vi "WPI_DashboardNTL FF to New Position2.vi"(7 "Version":i32=2, 8 "VI Refnum":refnum<vi>, 10 "TimeOffset (s)":dbl, 11 "Byte Stream File in":refnum<file>) -> (0 "Strings":T1, 1 "Unchanged":bool, 2 "New time (s)":dbl, 3 "Byte Stream File out":refnum<file>)   [LabVIEW 2025]
uses:
  <vilib>/Rock Robotics/WPI/Dashboard/WPI_DashboardLoggingRecord.ctl
  <vilib>/Rock Robotics/WPI/Dashboard/WPI_DashboardLogging Global.vi
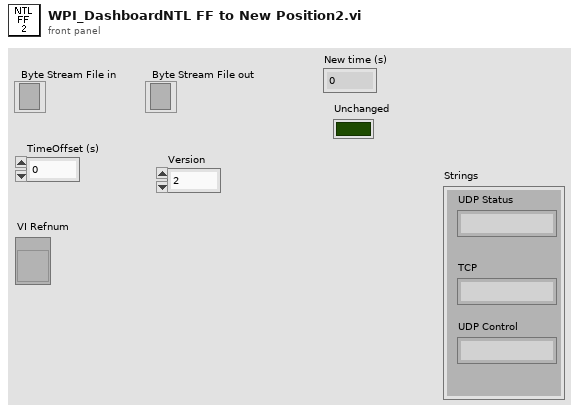
[diagram p1: front panel]
types:
  T1 = cluster{"UDP Status":string, "TCP":string, "UDP Control":string}
  T2 = typedef "WPI_DashboardLoggingRecord.ctl" = cluster{"time Ofst":i32, "video index":i32, "video index 2":i32, "video index 3":i32, "video index 4":i32, "UDP Status":string, "TCP":string, "UDP Control":string, "NT Updates":variant[]}
  T3 = cluster{"video index":i32, "video index 2":i32, "video index 3":i32, "video index 4":i32}
  T4 = cluster{"Video 1":i32, "Video 2":i32, "Video 3":i32, "Video 4":i32}
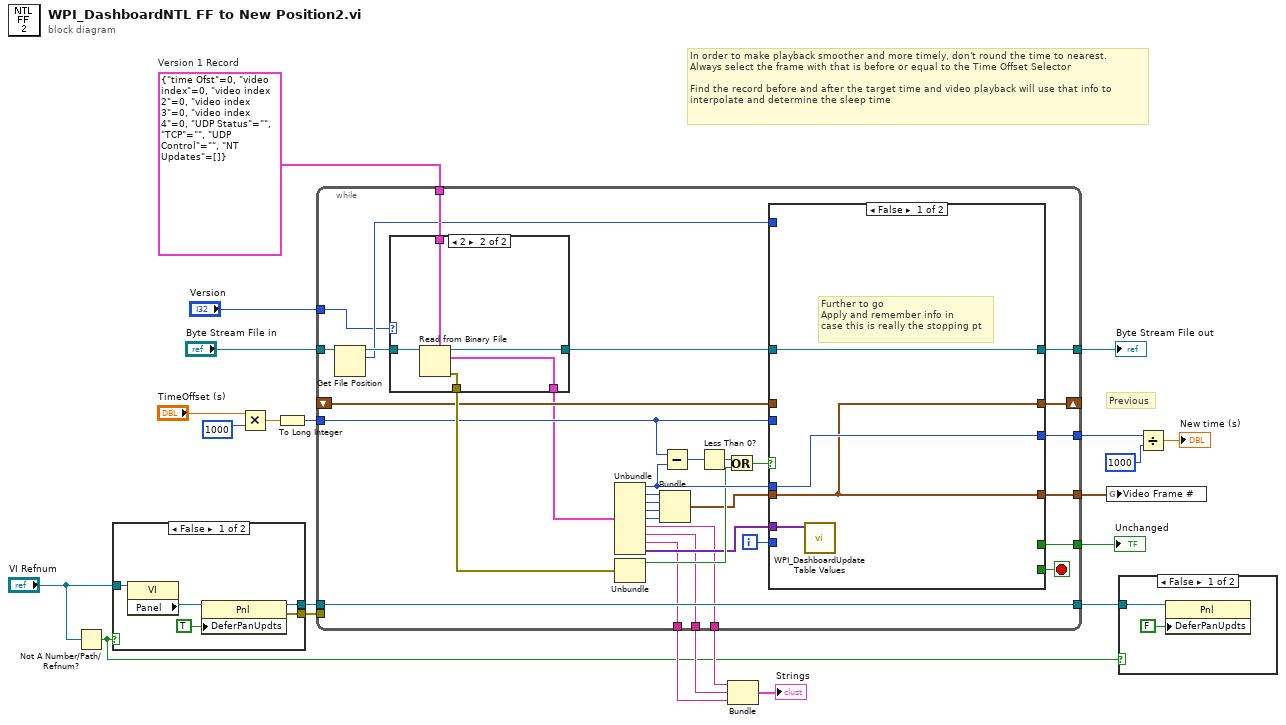
[diagram p0: block diagram]
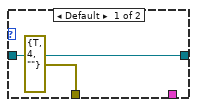
[diagram p4: hidden frame]
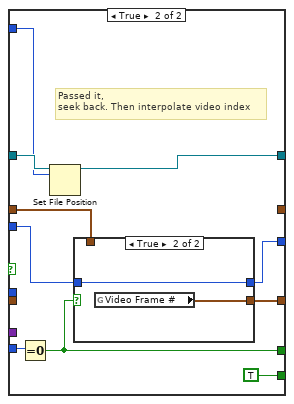
[diagram p5: hidden frame]
diagram:
  w4 = T2 {"time Ofst"=0, "video index"=0, "video index 2"=0, "video index 3"=0, "video index 4"=0, "UDP Status"="", "TCP"="", "UDP Control"="", "NT Updates"=[]}  # Version 1 Record
  # "Previous"
  # "In order to make playback smoother and more timely, don't round the time to nearest.\nAlways select the frame with that is before or equal to the Time Offset Selector\n\nFind the record before and after the target time and video playback will use that info to\ninterpolate and determine the sleep time"
  n1 = Not A Number/Path/Refnum?(number/path/refnum="VI Refnum") -> (NaN/Path/Refnum?=w1:bool)
  n2 = case shown="False" w1 {
    tunnel: [w25 _] -> w10
    tunnel: [w24 _] -> w9
    tunnel: "VI Refnum" -> [w23 _]
    frame False {
      n3 = property class="VI"(reference=w23) -> ("Panel"=w27:refnum<vi>)  [unwired: 1 in, 2 out]
      n4 = property class="Pnl"(reference=w27, "DeferPanUpdts"=TRUE ("Defer Panel Updates")) -> (reference out=w25:refnum<vi>, error out=w24:errorcluster)  [unwired: 1 in]
    }
    frame True {
    }
  }
  n5 = Multiply(x="TimeOffset (s)", y=1000) -> (x*y=w17:dbl)
  n6 = To Long Integer(number=w17) -> (32bit integer=w16:i32)
  n7 = while {
    tunnel: w4 -> [w59]
    tunnel: "Byte Stream File in" -> [w46]
    tunnel: [w56] -> w21
    tunnel: w16 -> [w52]
    shift-right: [w55] -> _
    shift-left: _ -> [w54]
    tunnel: [w50] -> w20
    tunnel: [w48] -> w13
    tunnel: [w47] -> w12
    tunnel: [w34] -> w8
    tunnel: [w36] -> w7
    tunnel: w10 -> [w38]
    tunnel: [w38] -> w11
    tunnel: w9 -> [_]
    tunnel: [w35] -> w6
    tunnel: "Version" -> [w28]
    i -> [w49]
    stop <- w39 stop-if-true
    n8 = Get File Position(7:w46) -> (2:w44:i64, 3:w45:refnum<file>)  [unwired: 1 in, 1 out]
    n9 = case shown="2" w28 {
      tunnel: w59 -> [_ w66]
      tunnel: [errorcluster {"status"=TRUE, "code"=4, "source"=""} ("error constant") w65] -> w58
      tunnel: [w60 w64] -> w57
      tunnel: [_ w63] -> w51
      tunnel: w45 -> [w60 w62]
      frame Default {
      }
      frame 2 {
        n10 = Read from Binary File(5:w66, 11:w62) -> (0:w65:errorcluster, 2:w63:T2, 3:w64:refnum<file>)  [unwired: 4 in, 1 out]
      }
    }
    n11 = Unbundle(w51) -> ("time Ofst"=w53:i32, "video index"=w33:i32, "video index 2"=w32:i32, "video index 3"=w31:i32, "video index 4"=w30:i32, "UDP Status"=w34:string, "TCP"=w35:string, "UDP Control"=w36:string, "NT Updates"=w37:variant[])
    n12 = Unbundle(w58) -> ("status"=w40:bool)  [unwired: 2 out]
    n13 = Bundle("video index"=w33, "video index 2"=w32, "video index 3"=w31, "video index 4"=w30) -> (w29:T3)  [unwired: 1 in]
    n14 = Subtract(x=w52, y=w53) -> (x-y=w41:i32)
    n15 = Less Than 0?(x=w41) -> (x < 0?=w43:bool)
    n16 = Or(x=w43, y=w40) -> (x .or. y?=w42:bool)
    n17 = case shown="False" w42 {
      tunnel: w57 -> [w69 w79]
      tunnel: [w69 w78] -> w56
      tunnel: [w67 _] -> w55
      tunnel: w54 -> [_ w71]
      tunnel: [_ TRUE] -> w39
      tunnel: w53 -> [w70 _]
      tunnel: w52 -> [_ w72]
      tunnel: w37 -> [w68 _]
      tunnel: [w70 w74] -> w50
      tunnel: w49 -> [_ w77]
      tunnel: [_ w73] -> w48
      tunnel: w29 -> [w67 _]
      tunnel: [w67 w75] -> w47
      tunnel: w44 -> [_ w76]
      frame False {
        # "Further to go\nApply and remember info in\ncase this is really the stopping pt"
        n18 = call <vilib>:"WPI_DashboardUpdate Table Values.vi"("Data Values"=w68) -> ()  [unwired: 11 in]
      }
      frame True {
        # "Passed it,\nseek back. Then interpolate video index"
        n19 = Equal To 0?(x=w77) -> (x = 0?=w73:bool)
        n20 = Set File Position(offset (in bytes) (0)=w76, refnum=w79) -> (refnum out=w78:refnum<file>)  [unwired: 2 in, 1 out]
        n21 = case shown="True" w73 {
          tunnel: [w82 w83] -> w75
          tunnel: w71 -> [w82 _]
          tunnel: [w81 w84] -> w74
          tunnel: w72 -> [w81 w84]
          frame False {
          }
          frame True {
            n22 = global read "WPI_DashboardLogging Global.vi" "Video Frame #"() -> (w83:T4)
          }
        }
      }
    }
  }
  "Byte Stream File out" <- w21
  "Unchanged" <- w13
  n23 = Bundle("UDP Status"=w8, "TCP"=w6, "UDP Control"=w7) -> (→"Strings":T1)  [unwired: 1 in]
  n24 = global write "WPI_DashboardLogging Global.vi" "Video Frame #"(w12) -> ()
  n25 = case shown="False" w1 {
    tunnel: w11 -> [w85 _]
    frame False {
      n26 = property class="Pnl"(reference=w85, "DeferPanUpdts"=FALSE ("Defer Panel Updates")) -> ()  [unwired: 1 in, 2 out]
    }
    frame True {
    }
  }
  n27 = Divide(x=w20, y=1000) -> (x/y=→"New time (s)":dbl)
